vi "Forward Kinematics View.vi"(10 "Joints":T2(array[cluster])=[{"Theta"=0.0, "d"=0.0, "a"=0.0, "alpha (degrees)"=0.0}] {"alpha (degrees)" format="%.2f"; "a" format="%.2f"; "d" scale=0.0..0.5; "Theta" scale=-180.0..180.0}, 11 "start pose":T1=[[1.0, 0.0, 0.0, 0.0], [0.0, 1.0, 0.0, 0.0], [0.0, 0.0, 1.0, 0.0], [0.0, 0.0, 0.0, 1.0]]) -> (2 "3D Picture":refnum<vi>(3d-picture), 3 "end effector pose":T1=[[1.0, 0.0, 0.0, 0.0], [0.0, 6.123233995736766e-17, 1.0, 0.0], [0.0, -1.0, 6.123233995736766e-17, 0.0], [0.0, 0.0, 0.0, 1.0]] format="%#_2g")   [LabVIEW 2024]
uses:
  <vilib>/Analysis/Matrix/Datatypes/RealMatrix.ctl
  <vilib>/Utility/miscctls.llb/LV3DPointTypeDef.ctl
  <vilib>/Analysis/Matrix/NI_Matrix.lvlib
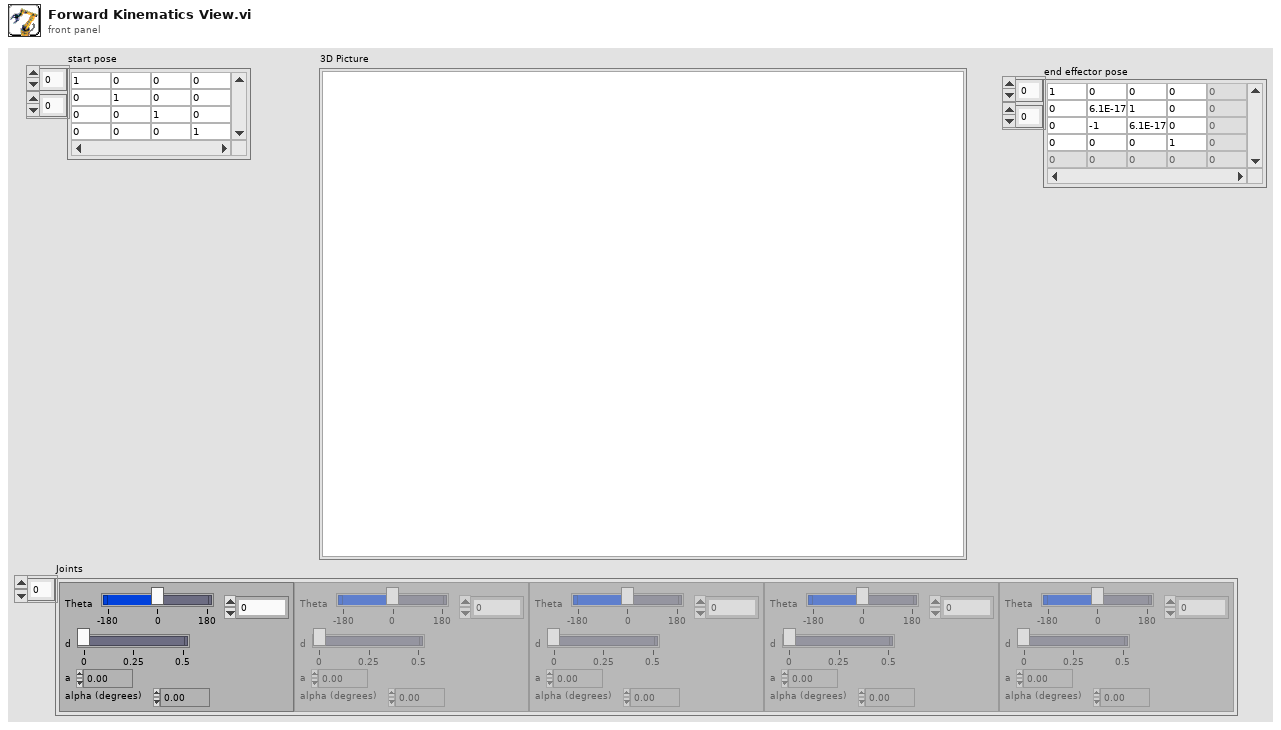
[diagram p1: front panel]
types:
  T1 = typedef "NI_Matrix.lvlib/RealMatrix.ctl" = dbl[][]
  T2 = cluster{"Theta":dbl, "d":dbl, "a":dbl, "alpha (degrees)":dbl}[]
  T3 = typedef "LV3DPointTypeDef.ctl" = cluster{"X":sgl, "Y":sgl, "Z":sgl}
  T4 = cluster{"Line width":sgl, "Line Color":u32, "Axes?":bool}
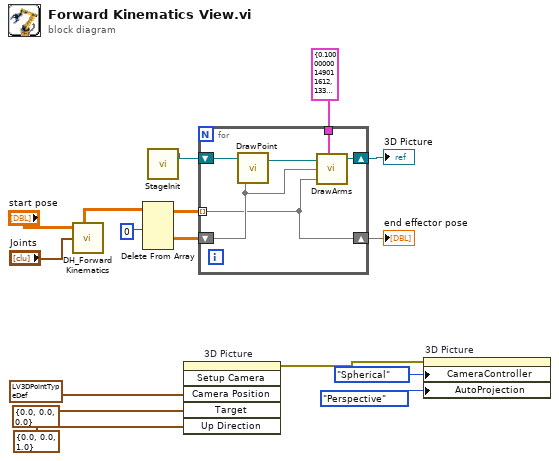
[diagram p0: block diagram]
diagram:
  n1 = call <userlib>:"DH_Forward Kinematics.vi"("start pose"="start pose", "Joints"="Joints") -> ("Intermediate Poses"=w4:dbl[][][])  [unwired: 2 in, 3 out]
  n2 = Delete From Array(array=w4, index (dim 0)=0 ("length")) -> (deleted portion=w1:dbl[][], array with subset deleted=w3:dbl[][][])  [unwired: 3 in]
  n3 = call <userlib>:"StageInit.vi"() -> ("Stage out"=w16:refnum<vi>)  [unwired: 4 in, 1 out]
  n4 = invoke on="3D Picture" class="SceneGraphDisp (strict)" method="Setup Camera"("Camera Position"=T3 {"X"=1.0, "Y"=1.0, "Z"=0.1}, "Target"=cluster{"X":sgl, "Y":sgl, "Z":sgl} {"X"=0.0, "Y"=0.0, "Z"=0.0}, "Up Direction"=cluster{"X":sgl, "Y":sgl, "Z":sgl} {"X"=0.0, "Y"=0.0, "Z"=1.0}) -> (error out=w12:errorcluster)  [unwired: 3 in, 5 out]
  n5 = for {
    shift-right: [w17] -> w14
    shift-left: w1 -> [w18]
    tunnel: T4 {"Line width"=0.1, "Line Color"=13354149, "Axes?"=TRUE} ("Params") -> [w22]
    shift-right: [w21] -> w13
    shift-left: w16 -> [w20]
    tunnel: w3 -> [w17] mode=indexing
    n6 = call <userlib>:"DrawPoint.vi"("Start"=w18, "Stage in"=w20) -> ("Stage out"=w19:refnum<vi>)  [unwired: 1 in]
    n7 = call <userlib>:"DrawArms.vi"("Stage in"=w19, "Params"=w22, "Start"=w18, "End"=w17) -> ("Stage out"=w21:refnum<vi>)  [unwired: 2 in, 1 out]
  }
  "end effector pose" <- w14
  "3D Picture" <- w13
  n8 = property on="3D Picture" class="SceneGraphDisp (strict)"(error in=w12, "CameraController"=enum16{"None", "Spherical", "Flying"}."Spherical" ("Camera Controller"), "AutoProjection"=enum16{"None", "Perspective", "Orthographic"}."Perspective" ("Auto Projection Mode")) -> ()  [unwired: 1 in, 2 out]
